vi "Variant LUT for Queue Ref.vi"(6 "Command":T2, 8 "Error In":errorcluster, 10 "Queue Name":string, 11 "Queue Ref In":T1) -> (0 "Error Out":errorcluster, 3 "Queue Ref Out":T1)   [LabVIEW 2014, in "SLL QSM.lvlib"]
doc: "Variant LUT for Storing the Queue References of SLL Queue Based State Machines.\n\nThis is used instead of directly using LabVIEW's \"Obtain Queue\" function because, the Obtain Queue Function creates a new Queue Reference for every call."
uses:
  SLL QSM.lvlib
  Typedefs/Queue Reference.ctl
  Typedefs/Queue Type.ctl
  Typedefs/Variant LUT Command.ctl
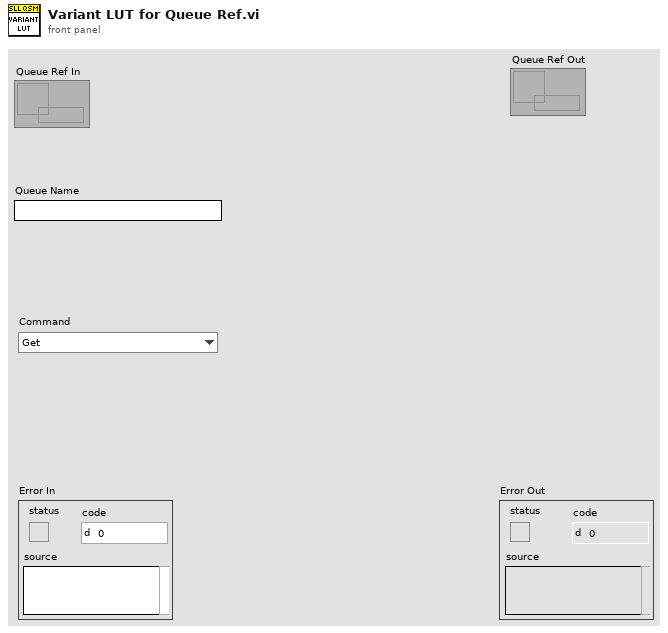
[diagram p1: front panel]
types:
  T1 = typedef "SLL QSM.lvlib/Queue Reference.ctl" = refnum<queue>
  T2 = typedef "SLL QSM.lvlib/Variant LUT Command.ctl" = enum16{"Get", "Set", "Delete"}
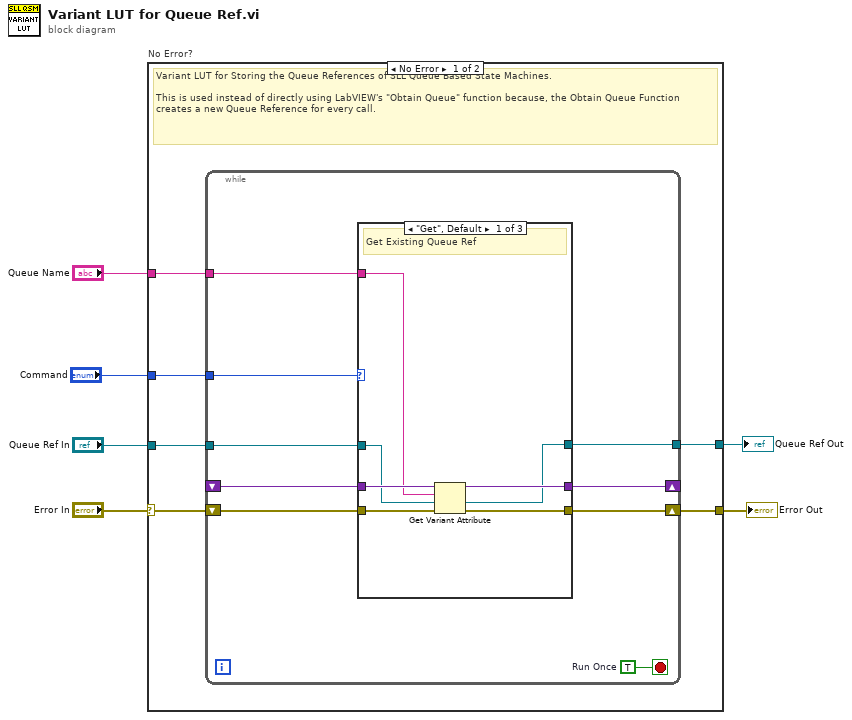
[diagram p0: block diagram]
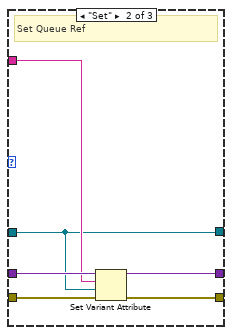
[diagram p2: hidden frame]
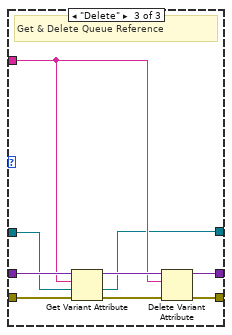
[diagram p3: hidden frame]
diagram:
  n1 = case "No Error?" shown="No Error" "Error In" {
    selector: "Error In" -> [w12 w45]
    tunnel: [w11 w45] -> w6
    tunnel: "Queue Name" -> [w9 _]
    tunnel: "Command" -> [w10 _]
    tunnel: "Queue Ref In" -> [w8 w44]
    tunnel: [w7 w44] -> w1
    frame No Error {
      # "Variant LUT for Storing the Queue References of SLL Queue Based State Machines.\n\nThis is used instead of directly using LabVIEW's \"Obtain Queue\" function because, the Obtain Queue Function creates a new Queue Reference for every call."
      n2 = while {
        tunnel: w10 -> [w19]
        shift-right: [w20] -> w11
        shift-left: w12 -> [w21]
        shift-right: [w17] -> _
        shift-left: _ -> [w16]
        tunnel: w9 -> [w15]
        tunnel: w8 -> [w14]
        tunnel: [w13] -> w7
        stop <- w18 stop-if-true
        w18 = TRUE  # Run Once
        n3 = case shown="\"Get\", Default" w19 {
          tunnel: w21 -> [w28 w34 w39]
          tunnel: [w27 w33 w43] -> w20
          tunnel: [w26 w31 w42] -> w17
          tunnel: w16 -> [w25 w32 w41]
          tunnel: w15 -> [w24 w30 w36]
          tunnel: w14 -> [w23 w29 w37]
          tunnel: [w22 w29 w35] -> w13
          frame "Get", Default {
            # "Get Existing Queue Ref"
            n4 = Get Variant Attribute(Variant=w25, name=w24, default value (empty Variant)=w23, error in=w28) -> (duplicate Variant=w26:variant, value=w22:T1, error out=w27:errorcluster)  [unwired: 1 out]
          }
          frame "Set" {
            # "Set Queue Ref"
            n5 = Set Variant Attribute(Variant=w32, name=w30, value=w29, error in=w34) -> (Variant out=w31:variant, error out=w33:errorcluster)  [unwired: 1 out]
          }
          frame "Delete" {
            # "Get & Delete Queue Reference"
            n6 = Get Variant Attribute(Variant=w41, name=w36, default value (empty Variant)=w37, error in=w39) -> (duplicate Variant=w40:variant, value=w35:T1, error out=w38:errorcluster)  [unwired: 1 out]
            n7 = Delete Variant Attribute(4:w38, 6:w36, 7:w40) -> (0:w43:errorcluster, 3:w42:variant)  [unwired: 1 out]
          }
        }
      }
    }
    frame Error {
    }
  }
  "Error Out" <- w6
  "Queue Ref Out" <- w1
